vi "ActorCoreEvent.vi"(8 "error in (no error)":errorcluster, 10 "ActorCoreMessage":string, 11 "HardwareSetup_modle001:HardwareSetup_modle001":refnum<class "HardwareSetup_model001.lvclass">) -> (0 "error out":errorcluster, 3 "HardwareSetup_modle001:HardwareSetup_modle001":refnum<class "HardwareSetup_model001.lvclass">)   [LabVIEW 2019, in "HardwareSetup_model001.lvlib" / "HardwareSetup_model001.lvclass"]
uses:
  HardwareSetup_model001.lvclass
  HardwareSetup_model001.lvclass/HardwareSetup_model001.ctl
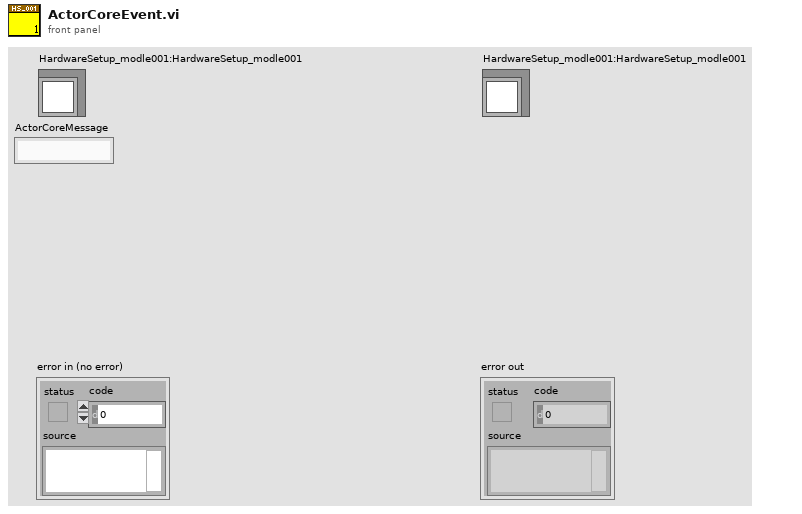
[diagram p1: front panel]
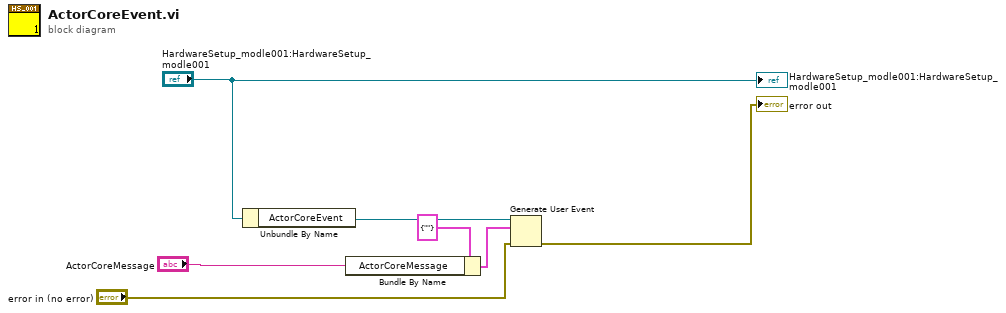
[diagram p0: block diagram]
diagram:
  n1 = Unbundle By Name("HardwareSetup_modle001:HardwareSetup_modle001") -> ("ActorCoreEvent"=w7:refnum<user-event>)
  n2 = Bundle By Name(cluster=cluster{"ActorCoreMessage":string} {"ActorCoreMessage"=""} ("event data"), "ActorCoreMessage"="ActorCoreMessage") -> (w5:cluster{"ActorCoreMessage":string})
  n3 = Generate User Event(user event=w7, event data cluster=w5, error in="error in (no error)") -> (error out=→"error out":errorcluster)  [unwired: 1 in, 1 out]
  "HardwareSetup_modle001:HardwareSetup_modle001" <- "HardwareSetup_modle001:HardwareSetup_modle001"
